vi "ReadStringImageAttribute.vi"(0 "device name":string, 1 "attribute name":string) -> (2 "value":string[][](array[string]), 3 "setpoint":string[][](array[string]), 4 "quality":i16, 5 "timestamp":dbl, 6 "success":bool=TRUE, 7 "error stack":string[](array[string]))   [LabVIEW 2014, in "tango.lvlib"]
uses:
  tango.lvlib
  Extractors/base/toStringImage.vi
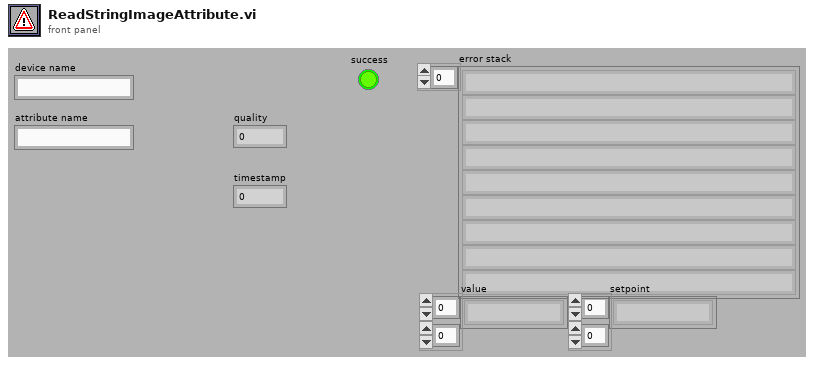
[diagram p1: front panel]
types:
  T1 = typedef "tango.lvlib/_AttributeQuality_t.ctl" = enum16{"VALID", "INVALID", "ALARM", "CHANGING", "UNKNOWN_QUALITY"}
  T2 = typedef "tango.lvlib/_AttributeDataType_t.ctl" = enum16{"STATE_SCA", "STATE_SPE", "STATE_IMG", "STRING_SCA", "STRING_SPE", "STRING_IMG", "BOOL_SCA", "BOOL_SPE", "BOOL_IMG", "UCHAR_SCA", "UCHAR_SPE", "UCHAR_IMG", "SHORT_SCA", "SHORT_SPE", "SHORT_IMG", "USHORT_SCA", "USHORT_SPE", "USHORT_IMG", "LONG_SCA", "LONG_SPE", "LONG_IMG", "ULONG_SCA", "ULONG_SPE", "ULONG_IMG", "LONG64_SCA", "LONG64_SPE", "LONG64_IMG", "ULONG64_SCA", "ULONG64_SPE", "ULONG64_IMG", "FLOAT_SCA", "FLOAT_SPE", "FLOAT_IMG", "DOUBLE_SCA", "DOUBLE_SPE", "DOUBLE_IMG", "UNKNOWN_DATA_TYPE"}
  T3 = cluster{"device name":string, "attribute name":string, "quality value":T1, "quality string":string, "timestamp":dbl, "dim. x":i32, "dim. y":i32, "value":u8[], "error code":i32, "error stack":string[], "data type":T2}[]
  T4 = cluster{"device name":string, "attribute name":string, "quality value":T1, "quality string":string, "timestamp":dbl, "dim. x":i32, "dim. y":i32, "value":u8[], "error code":i32, "error stack":string[], "data type":T2}
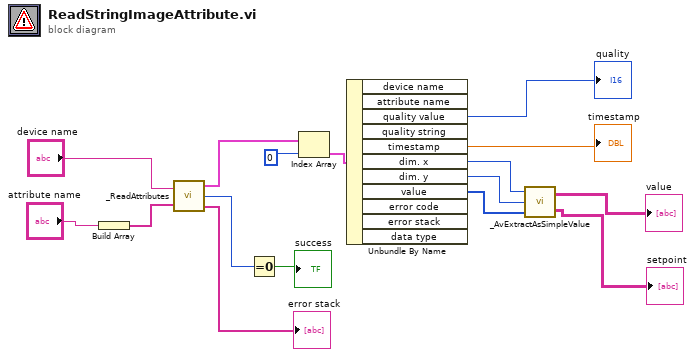
[diagram p0: block diagram]
diagram:
  n1 = Build Array("attribute name") -> (w8:string[])
  n2 = call "_ReadAttributes.vi"("device name"="device name", "attribute names"=w8) -> ("attribute values"=w10:T3, "error code"=w11:i32, "error stack"=→"error stack":string[])
  n3 = Equal To 0?(x=w11) -> (x = 0?=→"success":bool)
  n4 = Index Array(array=w10, index=0 ("indice")) -> (element=w13:T4)
  n5 = Unbundle By Name(w13) -> ("quality value"=→"quality":T1, "timestamp"=→"timestamp":dbl, "dim. x"=w5:i32, "dim. y"=w4:i32, "value"=w3:u8[])  [unwired: 6 out]
  n6 = call-poly "_AvExtractAsSimpleValue.vi"("value_in"=w3, "dim_y"=w4, "dim_x"=w5) -> ("setpoint"=→"setpoint":string[][], "value_out"=→"value":string[][])
